vi "Actor Core.vi"(8 "error in":errorcluster, 11 "SCHEMA_03 in":refnum<class "SCHEMA_03.lvclass">) -> (0 "error out":errorcluster, 3 "Actor out":refnum<class "Actor.lvclass">)   [LabVIEW 2020, in "SCHEMA_03.lvlib" / "SCHEMA_03.lvclass"]
doc: "(<B>Filename</B>: Actor Framework.lvlib:Actor.lvclass:Actor Core.vi)\n\nReceives messages to the actor, reacts to them, and initiates any error handling that may shut the actor down.\n\nDescendant classes may override this VI to append parallel tasks for the actor to complete while it handles messages. Overrides use the Call Parent Method node."
uses:
  SCHEMA_03.lvclass
  support/Actor Framework.lvlibp/1abvi3w/vi.lib/ActorFramework/Actor/Actor.lvclass
  D&C_SchemaBase/D&C_SchemaBase/D&C_SchemaBase.lvclass
panel:
  out "Source 1.T_31":dbl caption="Source 1.VAR 4" format="%#.3f"
  out "Source 1.T_16":dbl caption="Source 1.VAR 4" format="%#.3f"
  out "Source 2.pos_8":dbl(slide) caption="Source 2.Sinus" scale=-1.0..1.0
  out "Source 2.pos_7":dbl(slide) caption="Source 2.Sinus" scale=-1.0..1.0
  out "Source 2.pos_6":dbl(slide) caption="Source 2.Sinus" scale=-1.0..1.0
  out "Source 2.pos_5":dbl(slide) caption="Source 2.Sinus" scale=-1.0..1.0
  out "Source 2.pos_4":dbl(slide) caption="Source 2.Sinus" scale=-1.0..1.0
  out "Source 2.pos_3":dbl(slide) caption="Source 2.Sinus" scale=-1.0..1.0
  out "Source 2.pos_2":dbl(slide) caption="Source 2.Sinus" scale=-1.0..1.0
  out "Source 1.T_0":dbl caption="Random.VAR 1" format="%#.3f"
  out "Source 1.T_6":dbl caption="Source 1.VAR 4" format="%#.3f"
  out "Source 2.pos_1":dbl(slide) caption="Source 2.Sinus" scale=-1.0..1.0
  # "Les températures et le piston"
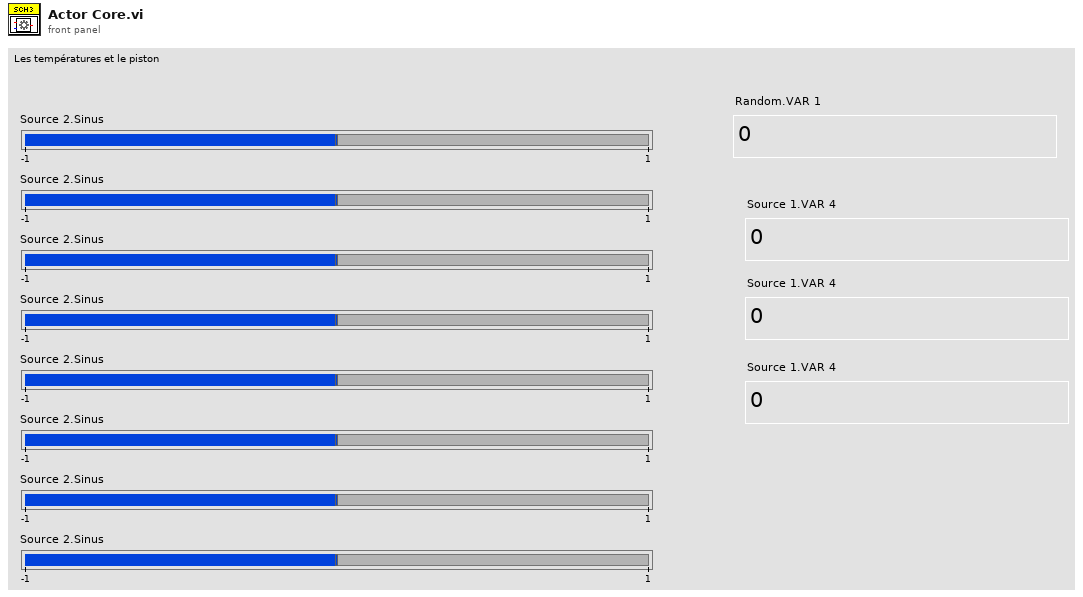
[diagram p1: front panel]
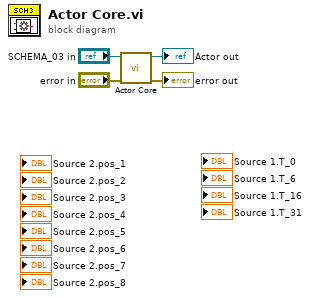
[diagram p0: block diagram]
diagram:
  n1 = call-parent "Actor Core.vi"("error in"="error in", "UI_Actor in"="SCHEMA_03 in") -> ("error out"=→"error out":errorcluster, "Actor out"=→"Actor out":refnum<class "Actor.lvclass">)  [unwired: 8 in]
